vi "Handle Error.vi"(8 "error in (no error)":errorcluster, 11 "Instrument in":refnum<class "Instrument.lvclass">) -> (0 "error out":errorcluster, 2 "Stop Process":bool, 3 "Instrument out":refnum<class "Instrument.lvclass">)   [LabVIEW 2017, in "Instrument.lvlib" / "Instrument.lvclass"]
uses:
  Instrument.lvclass
  <vilib>/TSS/ACRObat Test Framework/Classes/Base Objects/Acrobat Base Object/Acrobat Base Object/Acrobat Base Object.lvclass
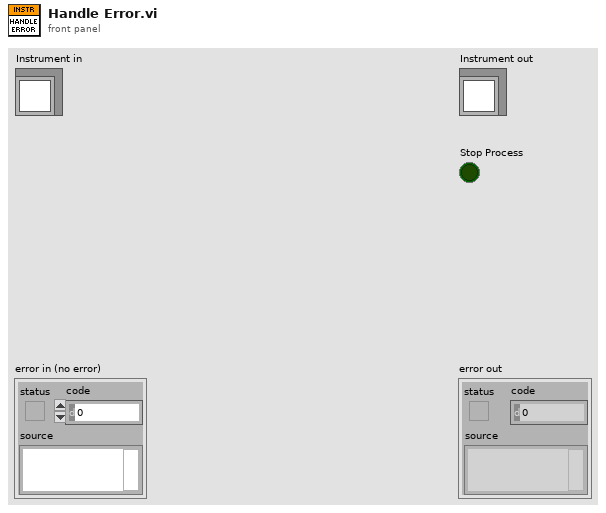
[diagram p1: front panel]
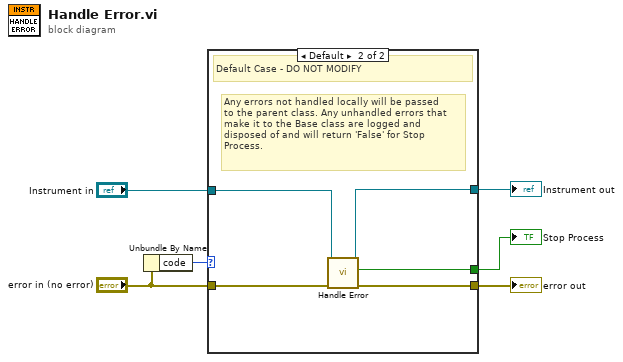
[diagram p0: block diagram]
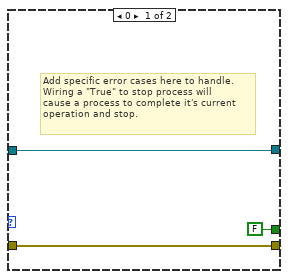
[diagram p2: hidden frame]
diagram:
  n1 = Unbundle By Name("error in (no error)") -> ("code"=w1:i32)
  n2 = case shown="Default" w1 {
    tunnel: [w8 w14] -> w6
    tunnel: [FALSE ("Stop Process") w13] -> w5
    tunnel: [w9 w12] -> w4
    tunnel: "error in (no error)" -> [w8 w11]
    tunnel: "Instrument in" -> [w9 w10]
    frame 0 {
      # "Add specific error cases here to handle.\nWiring a \"True\" to stop process will\ncause a process to complete it's current \noperation and stop."
    }
    frame Default {
      # "Any errors not handled locally will be passed\nto the parent class. Any unhandled errors that\nmake it to the Base class are logged and\ndisposed of and will return 'False' for Stop\nProcess."
      # "Default Case - DO NOT MODIFY"
      n3 = call-parent "Handle Error.vi"("error in (no error)"=w11, "Instrument in"=w10) -> ("error out"=w14:errorcluster, "Stop Process"=w13:bool, "Instrument out"=w12:refnum<class "Instrument.lvclass">)  [unwired: 7 in]
    }
  }
  "error out" <- w6
  "Instrument out" <- w4
  "Stop Process" <- w5
